vi "Write States.vi"(8 "error in (no error)":errorcluster, 10 "States":T1, 11 "GoToBallPlacementPositionTactic in":refnum<class "GoToBallPlacementPositionTactic.lvclass">) -> (0 "error out":errorcluster, 3 "GoToBallPlacementPositionTactic out":refnum<class "GoToBallPlacementPositionTactic.lvclass">)   [LabVIEW 2021, in "GoToBallPlacementPositionTactic.lvclass"]
uses:
  GoToBallPlacementPositionTactic.lvclass
  StatesGoToBallPlacementPositionTactic.ctl
  GoToBallPlacementPositionTactic.lvclass/GoToBallPlacementPositionTactic.ctl
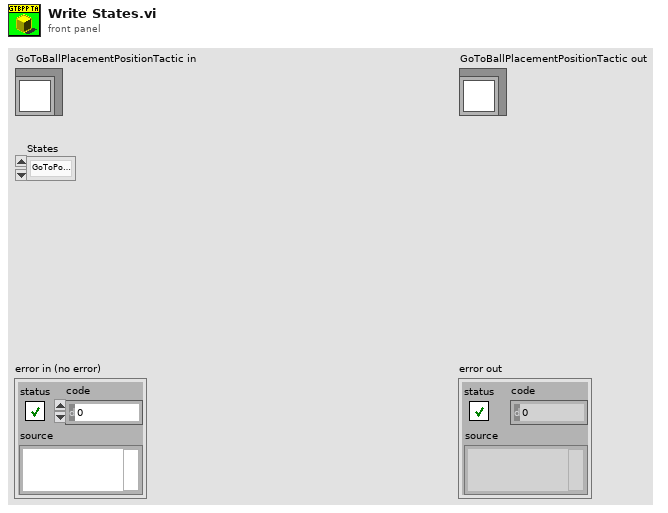
[diagram p1: front panel]
types:
  T1 = typedef "GoToBallPlacementPositionTactic.lvclass/StatesGoToBallPlacementPositionTactic.ctl" = enum16{"GoToPosition", "Exit"}
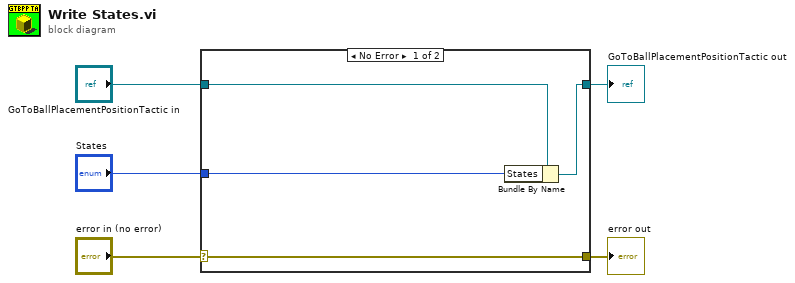
[diagram p0: block diagram]
diagram:
  n1 = case shown="No Error" "error in (no error)" {
    selector: "error in (no error)" -> [w9 w10]
    tunnel: [w9 w10] -> w4
    tunnel: [w7 w11] -> w2
    tunnel: "GoToBallPlacementPositionTactic in" -> [w8 w11]
    tunnel: "States" -> [w6 _]
    frame No Error {
      n2 = Bundle By Name(cluster=w8, "States"=w6) -> (w7:refnum<class "GoToBallPlacementPositionTactic.lvclass">)
    }
    frame Error {
    }
  }
  "error out" <- w4
  "GoToBallPlacementPositionTactic out" <- w2
